vi "Execute Query.vi"(8 "Error In":errorcluster, 10 "Table":string, 11 "Query":string) -> (0 "Error Out":errorcluster, 2 "Output Data":string[][](array[string]), 3 "Column Names":string[](array[string]))   [LabVIEW 2018, in "Database.lvlib"]
uses:
  Database.lvlib
  Action.ctl
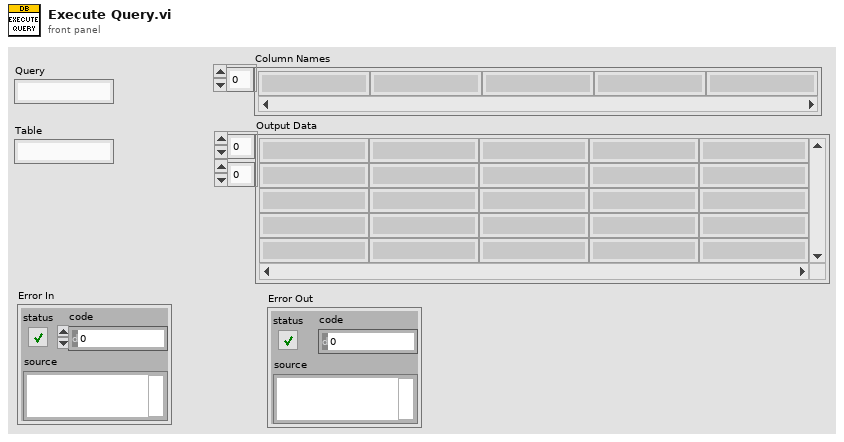
[diagram p1: front panel]
types:
  T1 = typedef "Database.lvlib/Action.ctl" = enum16{"Init", "List Tables", "List Columns", "Query", "Close"}
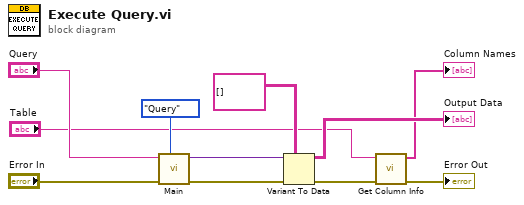
[diagram p0: block diagram]
diagram:
  n1 = call "Main.vi"("Action"=Action."Query", "Error In"="Error In", "Input"="Query") -> ("Error Out"=w2:errorcluster, "Output"=w9:variant)  [unwired: 7 in]
  n2 = Variant To Data(error in=w2, type=string[][] [], Variant=w9) -> (data=→"Output Data":string[][], error out=w1:errorcluster)
  n3 = call "Get Column Info.vi"("Error In"=w1, "Table"="Table") -> ("Error Out"=→"Error Out":errorcluster, "Column Names"=→"Column Names":string[])  [unwired: 7 in, 1 out]
